vi "Cmd-Rec Delete.vi"(4 "error in (no error)":errorcluster, 7 "command-recordset reference":T3) -> (0 "error out":errorcluster, 2 "recordset reference":T1, 3 "command reference":T2)   [LabVIEW 2017, in "NI_Database_API.lvlib"]
doc: "Destroys a <B>Command-Recordset</B> object created with a <B>Command-Recordset Create</B> VI."
uses:
  <vilib>/addons/database/NI_Database_API.lvlib
  <vilib>/addons/database/Command-Recordset.llb/Cmd-Rec Object Reference.ctl
  <vilib>/addons/database/Command.llb/Cmd ObjectReference.ctl
  <vilib>/addons/database/Recordset.llb/Rec ObjectReference.ctl
  <vilib>/Utility/_goopsup.llb/GOOP Object Repository Method.ctl
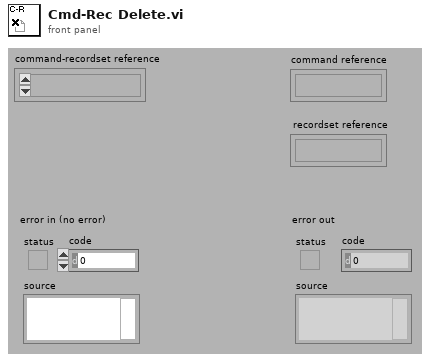
[diagram p1: front panel]
types:
  T1 = typedef "NI_Database_API.lvlib/Rec ObjectReference.ctl" = refnum<k1>
  T2 = typedef "NI_Database_API.lvlib/Cmd ObjectReference.ctl" = refnum<k1>
  T3 = typedef "NI_Database_API.lvlib/Cmd-Rec Object Reference.ctl" = refnum<k1>
  T4 = typedef "GOOP Object Repository Method.ctl" = enum16{"Create", "GetCopy", "GetModify", "Set", "Destroy", "Create Static", "Get All Refs", "Reset", "Get Statistics"}
  T5 = typedef "NI_Database_API.lvlib/Cmd-Rec Data Members.ctl" = cluster{"recordset reference":T1, "command reference":T2}
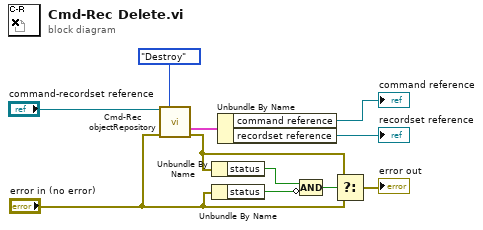
[diagram p0: block diagram]
diagram:
  n1 = call <vilib>:"Cmd-Rec objectRepository.vi"("command-recordset reference"="command-recordset reference", "method"=GOOP_Object_Repository_Method."Destroy", "error in (no error)"="error in (no error)") -> ("classDataOut"=w3:T5, "error out"=w9:errorcluster)  [unwired: 6 in, 5 out]
  n2 = Unbundle By Name(w9) -> ("status"=w8:bool)
  n3 = Unbundle By Name("error in (no error)") -> ("status"=w7:bool)
  n4 = Unbundle By Name(w3) -> ("command reference"=→"command reference":T2, "recordset reference"=→"recordset reference":T1)
  n5 = Compound Arithmetic op=AND(w8, invert w7) -> (w6:bool)
  n6 = Select(t=w9, s=w6, f="error in (no error)") -> (s? t:f=→"error out":errorcluster)
